vi "RegisterSweepRoutedMessage_Name.vi"() -> (1 "message name":string="EmsaDataEventCreator.RegisterSweep")   [LabVIEW 2017, in "EmsaDataEventCreator.lvlib"]
uses:
  <vilib>/addons/InsightCM/Devices/Shared/Emsa/EmsaDataEventCreator/EmsaDataEventCreator.lvlib
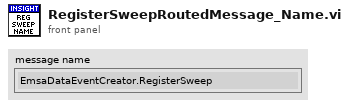
[diagram p1: front panel]
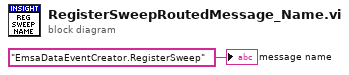
[diagram p0: block diagram]
diagram:
  "message name" <- "EmsaDataEventCreator.RegisterSweep"
